vi "ZMQ GEECS publisher.vi"() -> ()   [LabVIEW 2020]
uses:
  <vilib>/addons/zeromq/socket_type.ctl
  <vilib>/addons/zeromq/zmq_context.lvclass
  <vilib>/addons/zeromq/zmq_socket.lvclass
  <vilib>/addons/zeromq/zeromq.lvlib
panel:
  in  "endpoint":string="tcp://192.168.14.15:" caption="endpoint (publisher IP)"
  in  "port":i32=5555
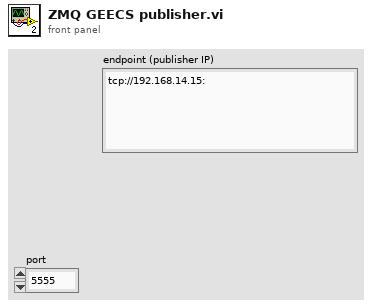
[diagram p1: front panel]
types:
  T1 = typedef "zeromq.lvlib/socket_type.ctl" = enum8{"ZMQ_PAIR", "ZMQ_PUB", "ZMQ_SUB", "ZMQ_REQ", "ZMQ_REP", "ZMQ_DEALER", "ZMQ_ROUTER", "ZMQ_PULL", "ZMQ_PUSH", "ZMQ_XPUB", "ZMQ_XSUB", "ZMQ_STREAM", "ZMQ_SERVER", "ZMQ_CLIENT", "ZMQ_RADIO", "ZMQ_DISH", "ZMQ_GATHER", "ZMQ_SCATTER", "ZMQ_DGRAM"}
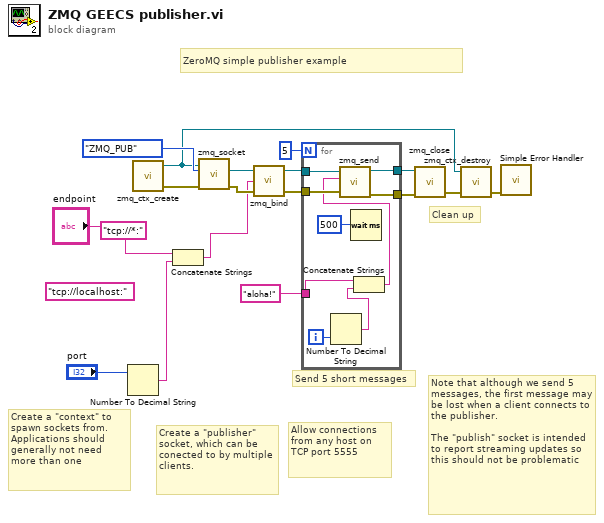
[diagram p0: block diagram]
diagram:
  (unwired) "tcp://localhost:" ("endpoint")
  (unwired) "tcp://*:" ("endpoint")
  # "ZeroMQ simple publisher example"
  # "Note that although we send 5 messages, the first message may be lost when a client connects to the publisher.\n\nThe \"publish\" socket is intended to report streaming updates so this should not be problematic"
  # "Clean up"
  # "Send 5 short messages"
  # "Allow connections from any host on TCP port 5555"
  # "Create a \"publisher\" socket, which can be conected to by multiple clients."
  # "Create a \"context\" to spawn sockets from. Applications should generally not need more than one"
  n1 = Number To Decimal String(number="port") -> (decimal integer string=w3:string)  [unwired: 1 in]
  n2 = call <vilib>:"zmq_ctx_create.vi"() -> ("error out"=w15:errorcluster, "context out"=w6:refnum<class "zmq_context.lvclass">)  [unwired: 4 in]
  n3 = Concatenate Strings("endpoint", w3) -> (w2:string)
  n4 = call <vilib>:"zmq_socket.vi"("error in"=w15, "socket type"=socket_type."ZMQ_PUB", "context in"=w6) -> ("error out"=w14:errorcluster, "socket out"=w5:refnum<class "zmq_socket.lvclass">)  [unwired: 2 in, 1 out]
  n5 = call <vilib>:"zmq_bind.vi"("error in"=w14, "endpoint"=w2, "socket in"=w5) -> ("error out"=w13:errorcluster, "socket out"=w17:refnum<class "zmq_socket.lvclass">)  [unwired: 1 in]
  n6 = for {
    N: 5 -> [_]
    tunnel: w17 -> [w26]
    tunnel: w13 -> [w25]
    tunnel: [w24] -> w12
    tunnel: "aloha!" ("format string") -> [w20]
    tunnel: [w22] -> w8
    i -> [w21]
    n7 = Number To Decimal String(number=w21) -> (decimal integer string=w18:string)  [unwired: 1 in]
    n8 = Wait (ms)(milliseconds to wait=u32 500) -> ()  [unwired: 1 out]
    n9 = Concatenate Strings(w20, w18) -> (w19:string)
    n10 = call <vilib>:"zmq_send.vi"("error in"=w25, "data"=w19, "socket in"=w26) -> ("error out"=w22:errorcluster, "socket out"=w24:refnum<class "zmq_socket.lvclass">)  [unwired: 4 in]
  }
  n11 = call <vilib>:"zmq_close.vi"("error in"=w8, "socket"=w12) -> ("error out"=w9:errorcluster)  [unwired: 3 in]
  n12 = call <vilib>:"zmq_ctx_destroy.vi"("error in"=w9, "context in"=w6) -> ("error out"=w10:errorcluster)  [unwired: 3 in]
  n13 = call <vilib>:"Simple Error Handler.vi"("error in (no error)"=w10) -> ()  [unwired: 4 in, 5 out]
